vi "string to timestamp.vi"(10 "is UTC (F)":bool, 11 "string":string) -> (3 "time stamp":timestamp)   [LabVIEW 2012]
uses:
  <vilib>/Utility/miscctls.llb/LVDateTimeRec.ctl
panel:
  out "Seconds":dbl
  out "Minute":i32
  out "Hour":i32
  out "Day":i32
  out "Month":i32
  out "Year":i32
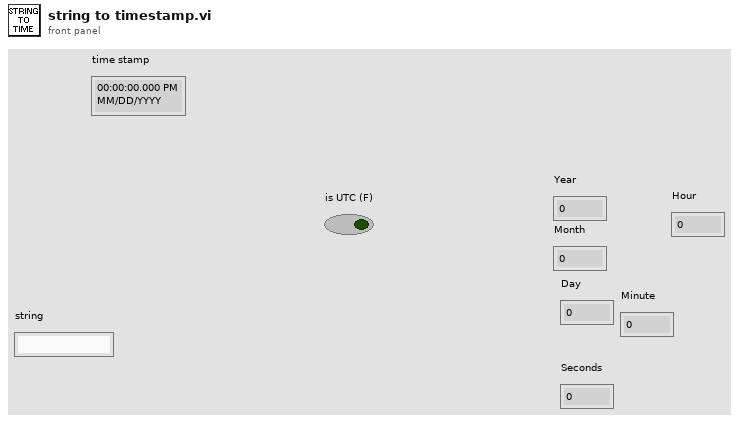
[diagram p1: front panel]
types:
  T1 = typedef "LVDateTimeRec.ctl" = cluster{"fractional second":dbl, "second":i32, "minute":i32, "hour":i32, "day of month":i32, "month":i32, "year":i32, "day of week":i32, "day of year":i32, "DST":i32}
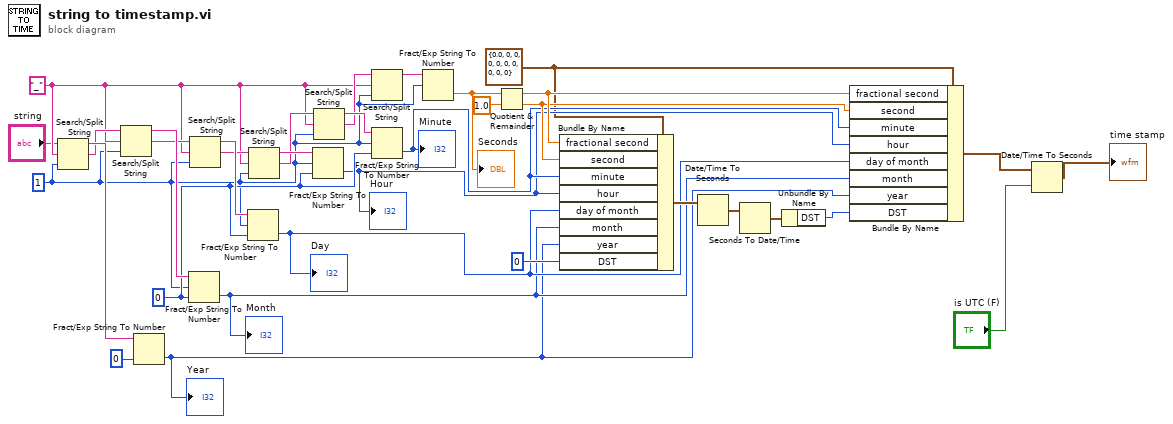
[diagram p0: block diagram]
diagram:
  w3 = T1 {"fractional second"=0.0, "second"=0, "minute"=0, "hour"=0, "day of month"=0, "month"=0, "year"=0, "day of week"=0, "day of year"=0, "DST"=0} ("date time rec")
  w20 = 1 ("offset (0)")
  w25 = 0 ("default (0 DBL)")
  w22 = "_" ("search string/char (-)")
  n1 = Search/Split String(string="string", search string/char (-)=w22, offset (0)=w20) -> (substring before match=w34:string, match + rest of string=w32:string)  [unwired: 1 out]
  n2 = Search/Split String(string=w32, search string/char (-)=w22, offset (0)=w20) -> (substring before match=w31:string, match + rest of string=w30:string)  [unwired: 1 out]
  n3 = Fract/Exp String To Number(string=w34, default (0 dbl)=0 ("default (0 DBL)")) -> (number=w5:i32)  [unwired: 2 in, 1 out]
  "Year" <- w5
  n4 = Fract/Exp String To Number(string=w31, offset=w20, default (0 dbl)=w25) -> (number=w6:i32)  [unwired: 1 in, 1 out]
  "Month" <- w6
  n5 = Search/Split String(string=w30, search string/char (-)=w22, offset (0)=w20) -> (substring before match=w29:string, match + rest of string=w27:string)  [unwired: 1 out]
  n6 = Fract/Exp String To Number(string=w29, offset=w20, default (0 dbl)=w25) -> (number=w7:i32)  [unwired: 1 in, 1 out]
  "Day" <- w7
  n7 = Search/Split String(string=w27, search string/char (-)=w22, offset (0)=w20) -> (substring before match=w28:string, match + rest of string=w24:string)  [unwired: 1 out]
  n8 = Fract/Exp String To Number(string=w28, offset=w20, default (0 dbl)=w25) -> (number=w8:i32)  [unwired: 1 in, 1 out]
  "Hour" <- w8
  n9 = Search/Split String(string=w24, search string/char (-)=w22, offset (0)=w20) -> (substring before match=w26:string, match + rest of string=w23:string)  [unwired: 1 out]
  n10 = Search/Split String(string=w23, search string/char (-)=w22, offset (0)=w20) -> (substring before match=w21:string)  [unwired: 2 out]
  n11 = Fract/Exp String To Number(string=w26, offset=w20, default (0 dbl)=w25) -> (number=w9:i32)  [unwired: 1 in, 1 out]
  "Minute" <- w9
  n12 = Fract/Exp String To Number(string=w21, offset=w20) -> (number=w19:dbl)  [unwired: 2 in, 1 out]
  "Seconds" <- w19
  n13 = Quotient & Remainder(x=w19, y=1.0) -> (x-y*floor(x/y)=w11:dbl, floor(x/y)=w10:dbl)
  n14 = Bundle By Name(cluster=w3, "fractional second"=w11, "second"=w10, "minute"=w9, "hour"=w8, "day of month"=w7, "month"=w6, "year"=w5, "DST"=0) -> (w17:T1)
  n15 = Date/Time To Seconds(2:w17) -> (0:w14:timestamp)  [unwired: 1 in]
  n16 = Seconds To Date/Time(time stamp (now)=w14) -> (date time rec=w13:T1)  [unwired: 1 in]
  n17 = Unbundle By Name(w13) -> ("DST"=w12:i32)
  n18 = Bundle By Name(cluster=w3, "fractional second"=w11, "second"=w10, "minute"=w9, "hour"=w8, "day of month"=w7, "month"=w6, "year"=w5, "DST"=w12) -> (w4:T1)
  n19 = Date/Time To Seconds(1:"is UTC (F)", 2:w4) -> (0:→"time stamp":timestamp)
